vi "Open Session.vi"(0 "FPGA Reference In":refnum<k20>, 5 "emulation model":T1=enum."PXIe-5172 (8CH - 410T)", 7 "adc clock rate (Hz)":dbl=250000000.0 format="%#_6p", 11 "error in":errorcluster) -> (4 "device session out":refnum<class "Device Session.lvclass">, 15 "error out":errorcluster)   [LabVIEW 2021, in "Device Session.lvclass"]
doc: "Opens a session to all bundled design libraries, including Register Bus, Multirecord Acquisition, Configuration, and Calibration, and initializes the scaling coefficients. This VI bundles these into a DVR session and wraps it with the session class wrapper.\n\n<B>Input Parameters</B>\n\n<B>fpga reference in</B> is the reference to the FPGA VI or bitfile of the RIO device specified. This parameter is obtained from the 'Open FPGA Reference' VI of this library.\n\n<B>emulation model</B> specifies the type of device that the config IDL will emulate, if FPGA emulation is enabled.\n\n<B>adc clock rate (Hz)</B> specifies the clock rate to use for the onboard clock when initializing clocking.\n\n<B>error in</B> describes error conditions that occur before this node runs. This input provides standard 'error in' functionality.\n\n<B>Output Parameters</B>\n\n<B>device session out</B> passes a reference to the session to the next VI.\n\n<B>error out</B> contains error information. This output provides standard 'error out' functionality."
uses:
  Device Session.lvclass
  <instrlib>/HSAI-RIO/Types/v1/Host/Typedefs/Model Name.ctl
  Private/Typedef/Device Session Object.ctl
  FPGA Refnum.ctl
  <instrlib>/_niInstr/FIFO Register Bus/v1/Host/niInstr FIFO Register Bus v1 Host.lvclass
  C:/Program Files (x86)/National Instruments/LabVIEW 2021/instr.lib/_niInstr/Instruction Framework/v1/Host/Instruction Target/niInstr Instruction Target v1 Host.lvclass
  <instrlib>/_niInstr/Instruction Framework/v1/Host/Subsystem Map/niInstr Subsystem Map v1 Host.lvclass
  <instrlib>/HSAI-RIO/Cal Data/Interface/v1/Host/Cal Data/niHSAI Cal Data v1 Host.lvclass
  <instrlib>/HSAI-RIO/Config/Group A/v1/Host/Main/niHSAI Group A Config v1 Host.lvclass
  C:/Program Files (x86)/National Instruments/LabVIEW 2021/instr.lib/HSAI-RIO/Config/Interface/v1/Host/niHSAI Config v1 Host.lvclass
  <instrlib>/_niInstr/Multirecord Acquisition/Interface/v1/Host/niInstr Multirecord Acquisition v1 Host.lvclass
  <instrlib>/HSAI-RIO/Types/v1/Host/Typedefs/Channel Configuration.ctl
  <instrlib>/HSAI-RIO/Types/v1/Host/Typedefs/Coupling.ctl
  <instrlib>/HSAI-RIO/Types/v1/Host/Typedefs/Impedance.ctl
  <instrlib>/HSAI-RIO/Types/v1/Host/Typedefs/Bandwidth.ctl
  <instrlib>/_niInstr/Multirecord Acquisition/Interface/v1/Host/Public/Scaling Coefficient.ctl
  Device Session.lvclass/Device Session.ctl
  <instrlib>/_niInstr/Multirecord Acquisition/Common/v1/Host/niInstr Multirecord Acquisition Common v1 Host.lvclass
  C:/Program Files (x86)/National Instruments/LabVIEW 2021/instr.lib/_niInstr/Multirecord Acquisition/Interface/v1/Host/niInstr Multirecord Acquisition v1 Host.lvclass
  <instrlib>/HSAI-RIO/Config/Interface/v1/Host/Protected/Configure ADC Clock For Onboard.vi
  <instrlib>/HSAI-RIO/Config/Interface/v1/Host/niHSAI Config v1 Host.lvclass
  <instrlib>/HSAI-RIO/Types/v1/Host/niHSAI Types v1 Host.lvlib
  C:/Program Files (x86)/National Instruments/LabVIEW 2021/instr.lib/HSAI-RIO/Config/Group A/v1/Host/Main/niHSAI Group A Config v1 Host.lvclass
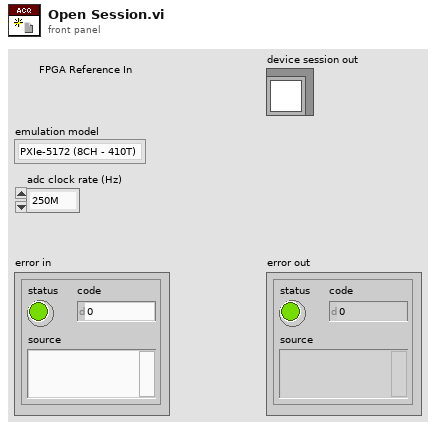
[diagram p1: front panel]
types:
  T1 = typedef "niHSAI Types v1 Host.lvlib/Model Name.ctl" = enum8{"None", "PXIe-5170R (4CH)", "PXIe-5170R (8CH)", "PXIe-5171R (8CH)", "PXIe-5172 (4CH - 325T)", "PXIe-5172 (8CH - 325T)", "PXIe-5172 (8CH - 410T)", "PXIe-5164", "PXIe-5163"}
  T2 = typedef "Device Session.lvclass/Device Session Object.ctl" = cluster{"fpga reference":T3, "reg bus":refnum<class "niInstr FIFO Register Bus v1 Host.lvclass">, "subsystem map":refnum<class "niInstr Subsystem Map v1 Host.lvclass">, "cal data":refnum<class "niHSAI Cal Data v1 Host.lvclass">, "config":refnum<class "niHSAI Group A Config v1 Host.lvclass">, "acquisition":refnum<class "niInstr Multirecord Acquisition v1 Host.lvclass">, "number of selected acq channels":u8, "selected acq channels":bool[], "number of channels":u32, "configured channels":bool[], "acq configuration":cluster{"number of samples":u64, "number of records":u64, "pretrigger samples":u64}, "actual channel configuration":T4[], "sample clock rate (Hz)":dbl, "scaling coefficients":T8[]}
  T3 = typedef "Device Session.lvclass/FPGA Refnum.ctl" = refnum<k20>
  T4 = typedef "niHSAI Types v1 Host.lvlib/Channel Configuration.ctl" = cluster{"channel":u32, "coupling":T5, "impedance":T6, "bandwidth":T7, "vertical range":dbl, "vertical offset":dbl}
  T5 = typedef "niHSAI Types v1 Host.lvlib/Coupling.ctl" = enum8{"Default", "DC", "AC"}
  T6 = typedef "niHSAI Types v1 Host.lvlib/Impedance.ctl" = enum8{"Default", "1 mega ohm", "50 ohm"}
  T7 = typedef "niHSAI Types v1 Host.lvlib/Bandwidth.ctl" = enum8{"Default", "Full Bandwidth", "Anti-alias Filter", "150 MHz"}
  T8 = typedef "niInstr Multirecord Acquisition v1 Host.lvclass/Scaling Coefficient.ctl" = cluster{"gain":dbl, "offset":dbl}
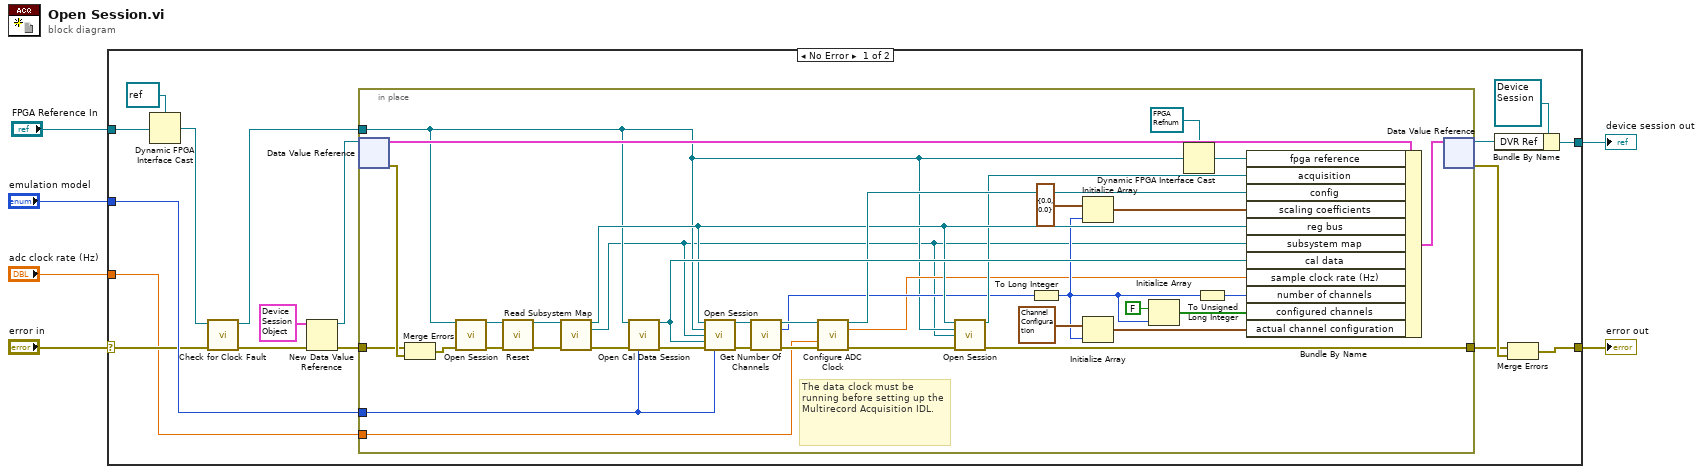
[diagram p0: block diagram]
diagram:
  n1 = case shown="No Error" "error in" {
    selector: "error in" -> [w13 w61]
    tunnel: [w16 w61] -> w5
    tunnel: [w22 _] -> w4
    tunnel: "FPGA Reference In" -> [w9 _]
    tunnel: "emulation model" -> [w14 _]
    tunnel: "adc clock rate (Hz)" -> [w7 _]
    frame No Error {
      n2 = Dynamic FPGA Interface Cast(Session In=refnum<k20> refnum ("fpga reference in"), Type=w9) -> (Session Out=w8:refnum<k20>)
      n3 = call "Check for Clock Fault.vi"("error in"=w13, "refnum in"=w8) -> ("error out"=w12:errorcluster, "refnum out"=w11:refnum<k20>)  [unwired: 8 in]
      n4 = New Data Value Reference(data value=T2 {"fpga reference"=refnum, "reg bus"=refnum, "subsystem map"=refnum, "cal data"=refnum, "config"=refnum, "acquisition"=refnum, "number of selected acq channels"=0, "selected acq channels"=[], "number of channels"=0, "configured channels"=[], "acq configuration"={"number of samples"=0, "number of records"=0, "pretrigger samples"=0}, "actual channel configuration"=[], "sample clock rate (Hz)"=0.0, "scaling coefficients"=[]} ("Cluster of class private data"), error in=w12) -> (data value reference=w19:refnum<data-value>, error out=w20:errorcluster)
      n5 = in-place {
        in-place-border: [w41] -> w17
        in-place-border: w20 -> [w53]
        in-place-border: w11 -> [w29]
        in-place-border: w14 -> [w39]
        in-place-border: w7 -> [w24]
        # "The data clock must be running before setting up the Multirecord Acquisition IDL."
        n6 = in-place-dvr #1(w19) -> (w55:T2, w54:errorcluster)
        n7 = Merge Errors(w53, w54) -> (w25:errorcluster)
        n8 = call <instrlib>:"Open Session.vi"("fpga ref"=w29, "error in"=w25) -> ("session out"=w60:refnum<class "niInstr FIFO Register Bus v1 Host.lvclass">, "error out"=w59:errorcluster)  [unwired: 12 in]
        n9 = call-dynamic "Reset.vi"("session in"=w60, "error in"=w59) -> ("session out"=w57:refnum<class "niInstr FIFO Register Bus v1 Host.lvclass">, "error out"=w58:errorcluster)  [unwired: 12 in]
        n10 = call <instrlib>:"Read Subsystem Map.vi"("instruction target in"=w57, "error in"=w58) -> ("instruction target out"=w43:refnum<class "niInstr FIFO Register Bus v1 Host.lvclass">, "subsystem map"=w26:refnum<class "niInstr Subsystem Map v1 Host.lvclass">, "error out"=w48:errorcluster)  [unwired: 11 in]
        n11 = call "Open Cal Data Session.vi"("fpga reference"=w29, "error in"=w48, "emulation model name"=w39) -> ("session out"=w49:refnum<class "niHSAI Cal Data v1 Host.lvclass">, "error out"=w56:errorcluster)  [unwired: 11 in]
        n12 = call <instrlib>:"Open Session.vi"("register bus in"=w43, "fpga interface in"=w29, "subsystem map in"=w26, "calibration data in"=w49, "error in"=w56, "emulation model name"=w39) -> ("session out"=w51:refnum<class "niHSAI Group A Config v1 Host.lvclass">, "error out"=w50:errorcluster)  [unwired: 8 in]
        n13 = call-dynamic "Get Number Of Channels.vi"("session in"=w51, "error in"=w50) -> ("session out"=w46:refnum<class "niHSAI Group A Config v1 Host.lvclass">, "number of channels"=w37:u32, "error out"=w47:errorcluster)  [unwired: 11 in]
        n14 = call-poly <instrlib>:"Configure ADC Clock.vi"("session in"=w46, "adc clock rate (Hz)"=w24, "error in"=w47) -> ("session out"=w45:refnum<class "niHSAI Group A Config v1 Host.lvclass">, "actual adc clock rate (Hz)"=w32:dbl, "error out"=w44:errorcluster)  [unwired: 8 in, 2 out]
        n15 = call <instrlib>:"Open Session.vi"("register bus"=w43, "fpga interface"=w29, "subsystem map"=w26, "error in"=w44) -> ("session out"=w42:refnum<class "niInstr Multirecord Acquisition Common v1 Host.lvclass">, "error out"=w41:errorcluster)  [unwired: 10 in]
        n16 = To Long Integer(number=w37) -> (32bit integer=w33:i32)
        n17 = Initialize Array(T8 {"gain"=0.0, "offset"=0.0} ("Scaling Coefficient"), w33) -> (w27:T8[])
        n18 = Initialize Array(T4 {"channel"=0, "coupling"=enum."Default", "impedance"=enum."Default", "bandwidth"=enum."Default", "vertical range"=0.0, "vertical offset"=0.0} ("channel configuration"), w33) -> (w36:T4[])
        n19 = Initialize Array(FALSE, w33) -> (w35:bool[])
        n20 = Dynamic FPGA Interface Cast(Session In=T3 refnum ("FPGA Interface"), Type=w29) -> (Session Out=w30:T3)
        n21 = To Unsigned Long Integer(number=w33) -> (unsigned 32bit integer=w34:u32)
        n22 = Bundle By Name(cluster=w55, "fpga reference"=w30, "acquisition"=w42, "config"=w45, "scaling coefficients"=w27, "reg bus"=w43, "subsystem map"=w26, "cal data"=w49, "sample clock rate (Hz)"=w32, "number of channels"=w34, "configured channels"=w35, "actual channel configuration"=w36) -> (w52:T2)
        n23 = in-place-dvr #1(w52) -> (w15:refnum<data-value>, w18:errorcluster)
      }
      n24 = Bundle By Name(cluster=refnum<class "Device Session.lvclass"> refnum ("ni5171R Session.lvclass"), "DVR Ref"=w15) -> (w22:refnum<class "Device Session.lvclass">)
      n25 = Merge Errors(w17, w18) -> (w16:errorcluster)
    }
    frame Error {
    }
  }
  "error out" <- w5
  "device session out" <- w4
